vi "exportKey2Str.vi"(0 "HGF_GPG in":refnum<class "HGF_GPG.lvclass">, 1 "options file":path, 2 "keyringfile":path, 3 "Sec keyringfile":path, 5 "error in (no error)":errorcluster, 6 "key-id":string, 7 "SecKey (f)":bool, 8 "Trust DB":path) -> (10 "dup Trust DB":path, 12 "dup key-id":string, 13 "success":bool, 14 "HGF_GPG out":refnum<class "HGF_GPG.lvclass">, 15 "dup options file":path, 16 "dup keyringfile":path, 17 "dup Sec keyringfile":path, 18 "Key":string, 19 "error out":errorcluster)   [LabVIEW 2012, in "HGF_GPG.lvlib" / "HGF_GPG.lvclass"]
doc: "Export a key to string. If no Key-ID is set, the Object's key will be returned in string."
uses:
  HGF_GPG.lvclass
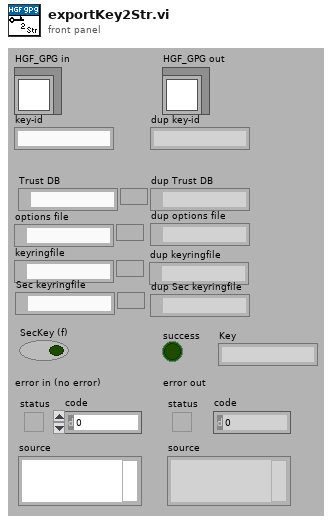
[diagram p1: front panel]
types:
  T1 = enum16{"list keys", "export", "import", "delete"}
  T2 = enum16{"open", "replace", "create", "open or create", "replace or create", "replace or create with confirmation"}
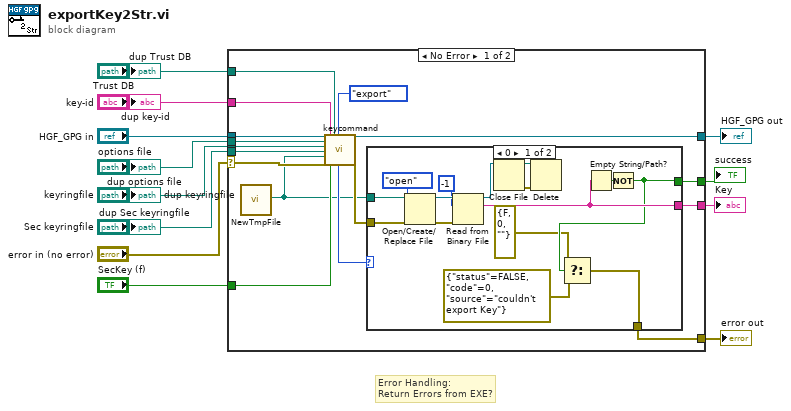
[diagram p0: block diagram]
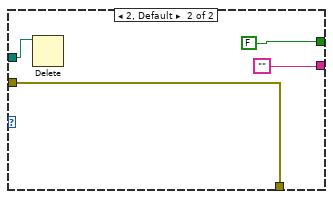
[diagram p2: hidden frame]
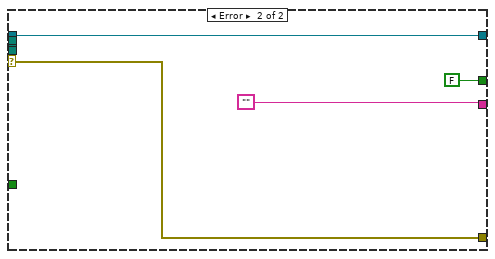
[diagram p3: hidden frame]
diagram:
  # "Error Handling:\nReturn Errors from EXE?"
  n1 = case shown="No Error" "error in (no error)" {
    selector: "error in (no error)" -> [w25 w51]
    tunnel: [w24 w51] -> w11
    tunnel: [w27 w50] -> w9
    tunnel: "HGF_GPG in" -> [w28 w50]
    tunnel: "key-id" -> [w16 _]
    tunnel: "SecKey (f)" -> [w20 _]
    tunnel: [w26 ""] -> w6
    tunnel: [w22 FALSE] -> w5
    tunnel: "keyringfile" -> [w18 _]
    tunnel: "options file" -> [w17 _]
    tunnel: "Sec keyringfile" -> [w15 _]
    tunnel: "Trust DB" -> [w14 _]
    frame No Error {
      n2 = call "NewTmpFile.vi"() -> ("path"=w19:path)  [unwired: 1 in, 18 out]
      n3 = call-dynamic "keycommand.vi"("HGF_GPG in"=w28, "options file"=w17, "keyringfile"=w18, "Sec keyringfile"=w15, "targetfile"=w19, "error in (no error)"=w25, "key-id"=w16, "SecKey (f)"=w20, "Trust DB"=w14, "Enum"=T1."export") -> ("return code"=w21:i32, "HGF_GPG out"=w27:refnum<class "HGF_GPG.lvclass">, "error out"=w23:errorcluster)  [unwired: 1 in, 14 out]
      n4 = case shown="0" w21 {
        tunnel: w19 -> [w43 w44]
        tunnel: [w33 ""] -> w26
        tunnel: [w30 w46] -> w24
        tunnel: w23 -> [w35 w46]
        tunnel: [w32 FALSE] -> w22
        frame 0 {
          n5 = Open/Create/Replace File(file path (use dialog)=w43, error in=w35, operation (0:open)=T2."open") -> (refnum out=w40:refnum<file>, error out=w41:errorcluster)  [unwired: 4 out]
          n6 = Read from Binary File(8:w41, 10:-1 ("count (1)"), 11:w40) -> (2:w33:string, 3:w38:refnum<file>)  [unwired: 5 out]
          n7 = Close File(refnum=w38) -> (path=w36:path, error out=w37:errorcluster)  [unwired: 1 in]
          n8 = Delete(path (use dialog)=w36, error in=w37) -> ()  [unwired: 6 out]
          n9 = Empty String/Path?(string/path=w33) -> (empty?=w34:bool)
          n10 = Not(x=w34) -> (.not. x?=w32:bool)
          n11 = Select(t=errorcluster {"status"=FALSE, "code"=0, "source"=""} ("error out"), s=w32, f=errorcluster {"status"=FALSE, "code"=0, "source"="couldn't export Key"}) -> (s? t:f=w30:errorcluster)
        }
        frame 2, Default {
          n12 = Delete(path (use dialog)=w44) -> ()  [unwired: 1 in, 6 out]
        }
      }
    }
    frame Error {
    }
  }
  "error out" <- w11
  "HGF_GPG out" <- w9
  "Key" <- w6
  "success" <- w5
  "dup keyringfile" <- "keyringfile"
  "dup key-id" <- "key-id"
  "dup options file" <- "options file"
  "dup Sec keyringfile" <- "Sec keyringfile"
  "dup Trust DB" <- "Trust DB"
